vi "ImgCtrl-Reset image ctrl.vi"(8 "error in":errorcluster) -> (0 "error out":errorcluster)   [LabVIEW 2020]
uses:
  Global variables/gl_Functional Imaging-Global variables.vi
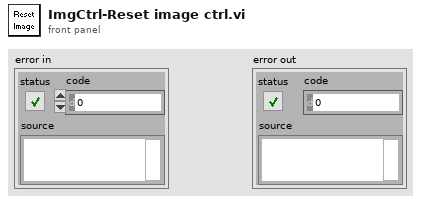
[diagram p1: front panel]
types:
  T1 = typedef "IMAQ Image.ctl" = refnum<image>
  T2 = typedef "Functional Imging UI Refs.ctl" = cluster{"Menu ref":refnum<k9>, "Image control":refnum<vi>, "VI ref":refnum<vi>, "XGrapher":refnum<vi>, "Smoothing":refnum<vi>, "POI Averaging":refnum<vi>, "Normalize":refnum<vi>, "POI data points in each trial":refnum<vi>, "Channel":refnum<vi>, "Experiment data folder path":refnum<vi>, "[ROI vis]":refnum<vi>, "[Groups] visbl":T3, "Group Name":refnum<vi>, "POI index":refnum<vi>, "Trial No.":refnum<vi>, "Intensity Zoom":refnum<vi>, "Trial Cursor Enabled":refnum<vi>, "Number of Trials (ind 1)":refnum<vi>, "Number of Trials (ind 2)":refnum<vi>, "MiniScans Available":refnum<vi>, "POI Available":refnum<vi>, "Defer graph updates":refnum<vi>, "Waveform selector":refnum<vi>, "#of selected POI":refnum<vi>, "#of selected MiniScans":refnum<vi>, "#of selected groups":refnum<vi>, "Max Z-Projection":refnum<vi>, "Z-Plane Selector":refnum<vi>, "Index of miniscan point to visualise":refnum<vi>, "ROI vis. mode":refnum<vi>, "Total # of points":refnum<vi>, "Index of group clicked on":refnum<vi>, "Pane 1":refnum<vi>, "Pane 2":refnum<vi>, "Pane 3":refnum<vi>, "Pane 4":refnum<vi>, "Pane 5":refnum<vi>, "Pane 6":refnum<vi>, "Deselect all ROI":refnum<vi>, "Deselect all groups":refnum<vi>}
  T3 = typedef "Groups array referecne.ctl" = refnum<vi>
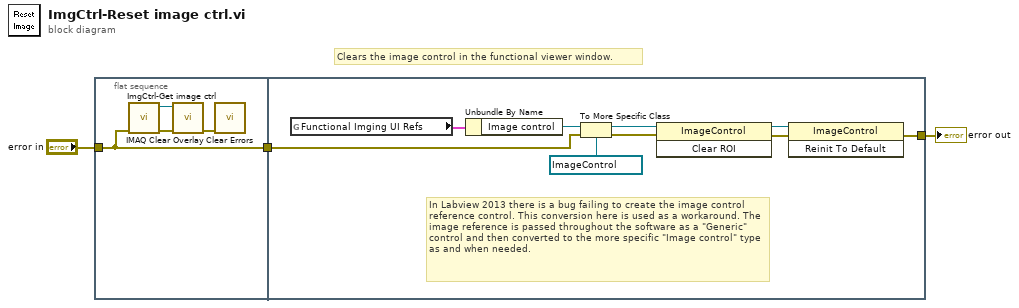
[diagram p0: block diagram]
diagram:
  # "Clears the image control in the functional viewer window."
  n1 = flat-sequence {
    tunnel: "error in" -> [w4]
    tunnel: [w4] -> w1
    tunnel: [w9] -> w3
    tunnel: w1 -> [w8]
    frame #0 {
      n2 = call "ImgCtrl-Get image ctrl.vi"("error in"=w4) -> ("error out"=w7:errorcluster, "Image"=w6:T1)  [unwired: 9 in]
      n3 = call "IMAQ Clear Overlay"("error in (no error)"=w7, "Image"=w6) -> ("error out"=w5:errorcluster)  [unwired: 8 in, 1 out]
      n4 = call <vilib>:"Clear Errors.vi"("error in (no error)"=w5) -> ()  [unwired: 5 in, 2 out]
    }
    frame #1 {
      # "In Labview 2013 there is a bug failing to create the image control reference control. This conversion here is used as a workaround. The image reference is passed throughout the software as a \"Generic\" control and then converted to the more specific \"Image control\" type as and when needed."
      n5 = global read "gl_Functional Imaging-Global variables.vi" "Functional Imging UI Refs"() -> (w15:T2)
      n6 = Unbundle By Name(w15) -> ("Image control"=w14:refnum<vi>)
      n7 = To More Specific Class(target class=refnum<vi> refnum ("Image"), reference=w14, error in=w8) -> (specific class reference=w12:refnum<vi>, error out=w10:errorcluster)
      n8 = invoke on="Invoke Node" class="ImageControl" method="Clear ROI"(reference=w12, error in=w10) -> (reference out=w13:refnum<vi>, error out=w11:errorcluster)  [unwired: 1 in, 1 out]
      n9 = invoke on="Invoke Node" class="ImageControl" method="Reinit To Default"(reference=w13, error in=w11) -> (error out=w9:errorcluster)  [unwired: 1 in, 2 out]
    }
  }
  "error out" <- w3
